vi "SN Sorter.vi"(0 "Run Screen SN":string, 5 "Specified SNs":string[](array[string]), 9 "Data":string[][](array[string]), 11 "Profile":string[][](array[string])) -> (4 "Next SN":string, 8 "Untested SNs":string[](array[string]), 15 "Tested SNs":string[](array[string]))   [LabVIEW 2013]
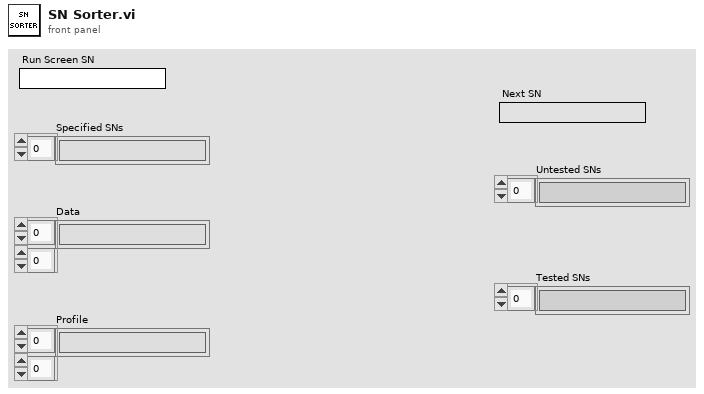
[diagram p1: front panel]
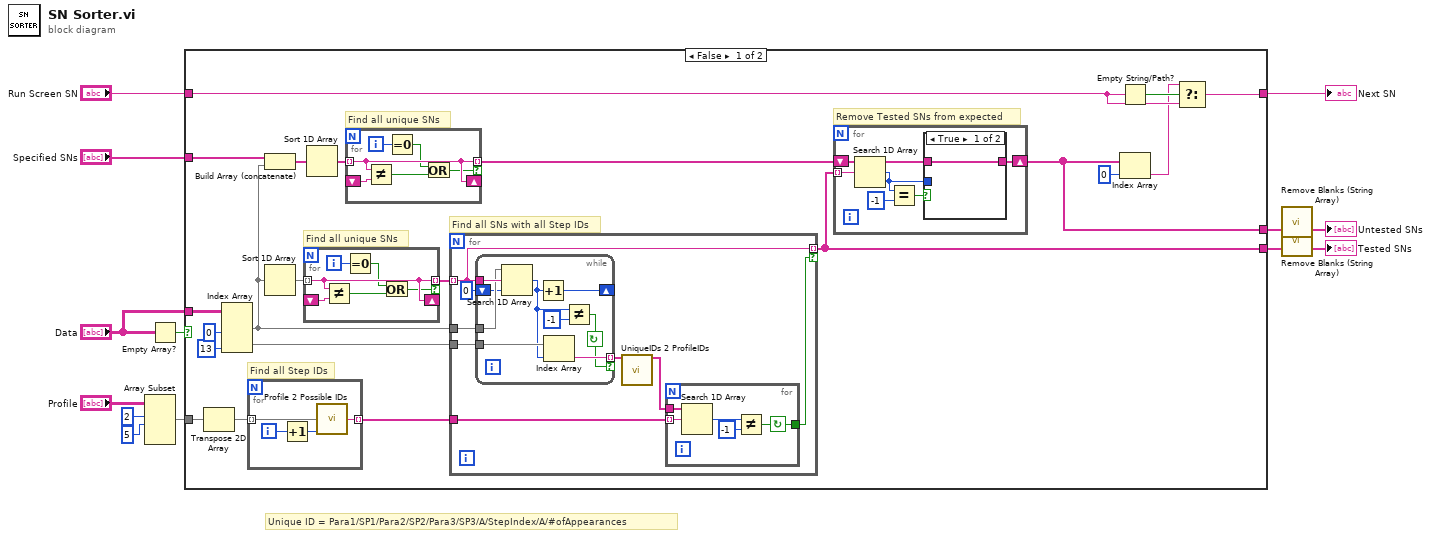
[diagram p0: block diagram]
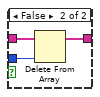
[diagram p2: hidden frame]
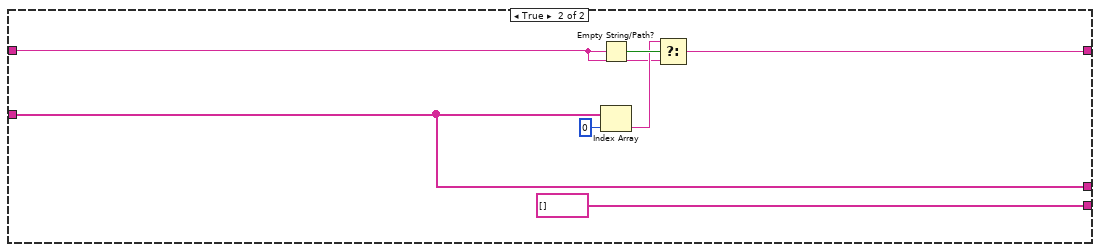
[diagram p3: hidden frame]
diagram:
  # "Unique ID = Para1/SP1/Para2/SP2/Para3/SP3/A/StepIndex/A/#ofAppearances"
  n1 = Array Subset(array="Profile", index (row)=2 ("index"), length (row)=5 ("length")) -> (w1:string[][])  [unwired: 2 in]
  n2 = Empty Array?(array="Data") -> (empty?=w13:bool)
  n3 = case shown="False" w13 {
    tunnel: "Specified SNs" -> [w24 w85]
    tunnel: "Run Screen SN" -> [w18 w83]
    tunnel: [w17 w84] -> w10
    tunnel: [w19 w85] -> w7
    tunnel: [w20 string[] [] ("Tested SNs")] -> w8
    tunnel: w1 -> [w34 _]
    tunnel: "Data" -> [w32 _]
    frame False {
      # "Remove Tested SNs from expected"
      # "Find all unique SNs"
      # "Find all SNs with all Step IDs"
      # "Find all Step IDs"
      # "Find all unique SNs"
      n4 = Transpose 2D Array(2D array=w34) -> (transposed array=w33:string[][])
      n5 = Index Array(array=w32, index (col) #1=0 ("disabled index (col)"), index (col) #2=13 ("index (col)")) -> (element #1=w25:string[], element #2=w29:string[])  [unwired: 2 in]
      n6 = for {
        tunnel: w33 -> [w82] mode=indexing
        tunnel: [w81] -> w26 mode=indexing
        i -> [w80]
        n7 = Increment(x=w80) -> (x+1=w79:i32)
        n8 = call "Profile 2 Possible IDs.vi"("Profile Step"=w82, "StepIndex"=w79) -> ("Step ID"=w81:string)  [unwired: 13 in]
      }
      n9 = Build Array (concatenate)(w24, w25) -> (w22:string[])
      n10 = Sort 1D Array(array=w25) -> (sorted array=w28:string[])
      n11 = for {
        tunnel: w28 -> [w55] mode=indexing
        shift-right: [w55] -> _
        shift-left: _ -> [w56]
        tunnel: [w55] -> w27 mode=indexing if=w53
        i -> [w54]
        n12 = Not Equal?(x=w55, y=w56) -> (x != y?=w52:bool)
        n13 = Equal To 0?(x=w54) -> (x = 0?=w51:bool)
        n14 = Or(x=w51, y=w52) -> (x .or. y?=w53:bool)
      }
      n15 = Sort 1D Array(array=w22) -> (sorted array=w23:string[])
      n16 = for {
        tunnel: w23 -> [w49] mode=indexing
        shift-right: [w49] -> _
        shift-left: _ -> [w50]
        tunnel: [w49] -> w21 mode=indexing if=w47
        i -> [w48]
        n17 = Not Equal?(x=w49, y=w50) -> (x != y?=w46:bool)
        n18 = Equal To 0?(x=w48) -> (x = 0?=w45:bool)
        n19 = Or(x=w45, y=w46) -> (x .or. y?=w47:bool)
      }
      n20 = for {
        tunnel: w25 -> [w64]
        tunnel: w29 -> [w63]
        tunnel: w27 -> [w60] mode=indexing
        tunnel: w26 -> [w61]
        tunnel: [w60] -> w20 mode=indexing if=w59
        n21 = while {
          tunnel: w60 -> [w78]
          tunnel: w64 -> [w77]
          tunnel: w63 -> [w74]
          shift-right: [w70] -> _
          shift-left: 0 -> [w76]
          tunnel: [w73] -> w58 mode=indexing if=w72
          stop <- w72 continue-if-true
          n22 = Search 1D Array(1D array=w77, element=w78, start index (0)=w76) -> (index of element=w71:i32)
          n23 = Increment(x=w71) -> (x+1=w70:i32)
          n24 = Index Array(array=w74, index=w71) -> (element=w73:string)
          n25 = Not Equal?(x=w71, y=-1) -> (x != y?=w72:bool)
        }
        n26 = call "UniqueIDs 2 ProfileIDs.vi"("Unique IDs"=w58) -> ("Profile IDs"=w57:string[])  [unwired: 14 in]
        n27 = for {
          tunnel: w61 -> [w68] mode=indexing
          tunnel: w57 -> [w69]
          tunnel: [w65] -> w59
          stop <- w65 continue-if-true
          n28 = Search 1D Array(1D array=w69, element=w68) -> (index of element=w67:i32)  [unwired: 1 in]
          n29 = Not Equal?(x=w67, y=-1) -> (x != y?=w65:bool)
        }
      }
      n30 = for {
        tunnel: w20 -> [w40] mode=indexing
        shift-right: [w36] -> w19
        shift-left: w21 -> [w38]
        n31 = Search 1D Array(1D array=w38, element=w40) -> (index of element=w35:i32)  [unwired: 1 in]
        n32 = Equal?(x=w35, y=-1) -> (x = y?=w37:bool)
        n33 = case shown="True" w37 {
          tunnel: w38 -> [w41 w44]
          tunnel: [w41 w43] -> w36
          tunnel: w35 -> [_ w42]
          frame True {
          }
          frame False {
            n34 = Delete From Array(array=w44, index=w42) -> (array with subset deleted=w43:string[])  [unwired: 1 in, 1 out]
          }
        }
      }
      n35 = Empty String/Path?(string/path=w18) -> (empty?=w16:bool)
      n36 = Index Array(array=w19, index=0) -> (element=w15:string)
      n37 = Select(t=w15, s=w16, f=w18) -> (s? t:f=w17:string)
    }
    frame True {
      n38 = Empty String/Path?(string/path=w83) -> (empty?=w88:bool)
      n39 = Index Array(array=w85, index=0) -> (element=w87:string)
      n40 = Select(t=w87, s=w88, f=w83) -> (s? t:f=w84:string)
    }
  }
  "Next SN" <- w10
  n41 = call "Remove Blanks (String Array).vi"("Array In"=w7) -> ("Array Out"=→"Untested SNs":string[])  [unwired: 18 in]
  n42 = call "Remove Blanks (String Array).vi"("Array In"=w8) -> ("Array Out"=→"Tested SNs":string[])  [unwired: 18 in]
